vi "create.OrderExecuted.vi"(11 "OrderExecuted.Parms":T1={"Time Offset"=457000, "Order Id"="ORID0001", "Executed\nQuantity"=200, "Execution Id"=0}) -> (2 "Bytes.Out":u8[](array[numeric]) format="%.0x", 3 "PitchMessage out":refnum<class "OrderExecuted.lvclass">)   [LabVIEW 2022 SP3]
uses:
  OrderExecuted/OrderExecuted.Parameters.ctl
  OrderExecuted/OrderExecuted.lvclass
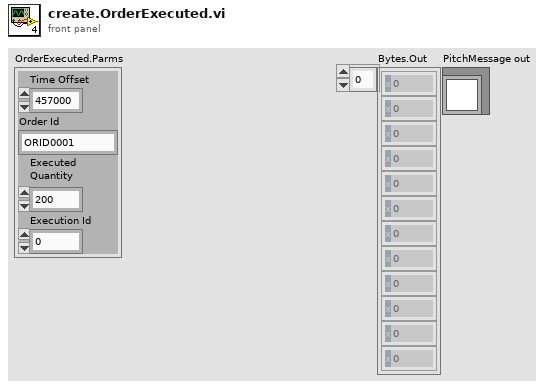
[diagram p1: front panel]
types:
  T1 = typedef "OrderExecuted.lvclass/OrderExecuted.Parameters.ctl" = cluster{"Time Offset":u32, "Order Id":string, "Executed\nQuantity":u32, "Execution Id":u64}
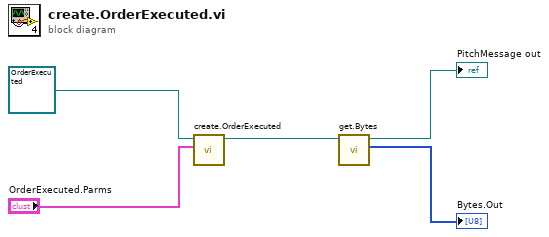
[diagram p0: block diagram]
diagram:
  n1 = call-dynamic "create.OrderExecuted.vi"("OrderExecuted.Parms"="OrderExecuted.Parms", "OrderExecuted in"=refnum<class "OrderExecuted.lvclass"> refnum ("OrderExecuted.lvclass")) -> ("OrderExecuted out"=w3:refnum<class "OrderExecuted.lvclass">)  [unwired: 8 in, 1 out]
  n2 = call-dynamic "get.Bytes.vi"("PitchMessage in"=w3) -> ("Bytes.Out"=→"Bytes.Out":u8[], "PitchMessage out"=→"PitchMessage out":refnum<class "OrderExecuted.lvclass">)  [unwired: 8 in, 1 out]
